vi "RMGetFrameCounters.vi"(0 "ResultManager":T1, 11 "error in (no error)":errorcluster) -> (3 "capturedFrames":i32, 4 "ResultManager (out)":T1, 6 "startFrame":i32, 8 "totalLocalizationsDone":i32, 10 "endFrame":i32, 13 "lostFrames":i32, 14 "lastSaveFrame":i32, 15 "error":errorcluster)   [LabVIEW 2011]
uses:
  ResultManagerInstance.ctl
  QTrkDLL.vi
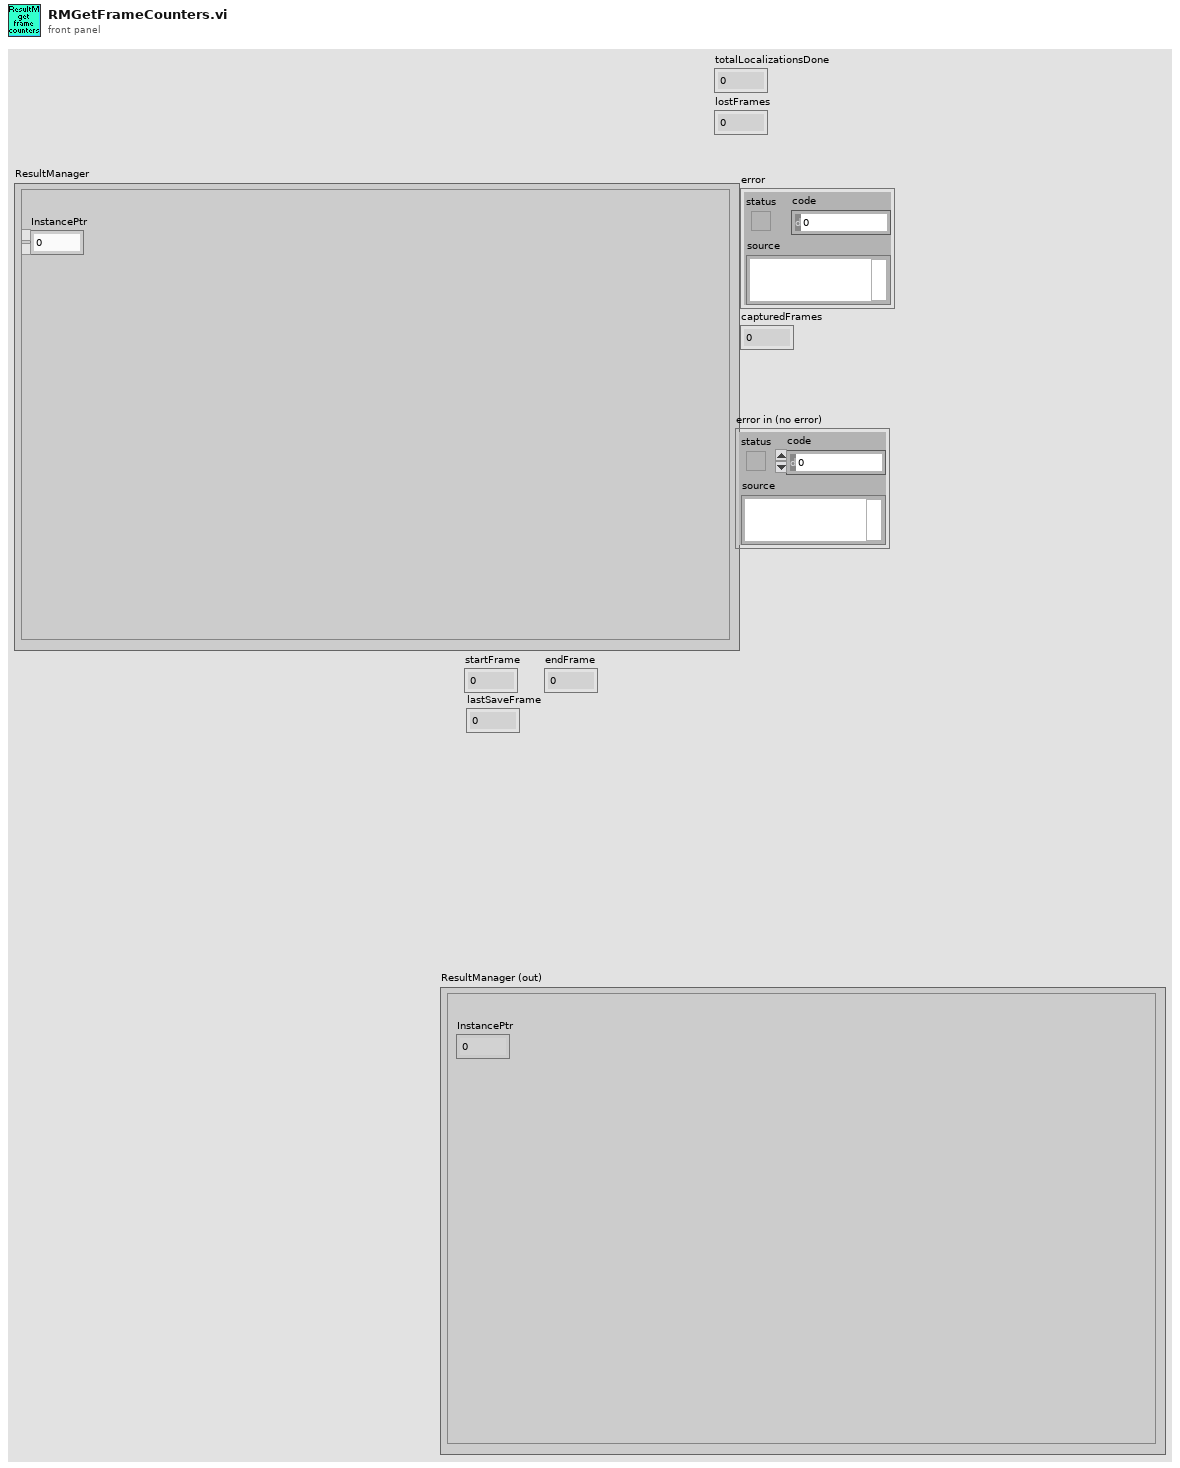
[diagram p1: front panel]
types:
  T1 = typedef "ResultManagerInstance.ctl" = cluster{"InstancePtr":u64}
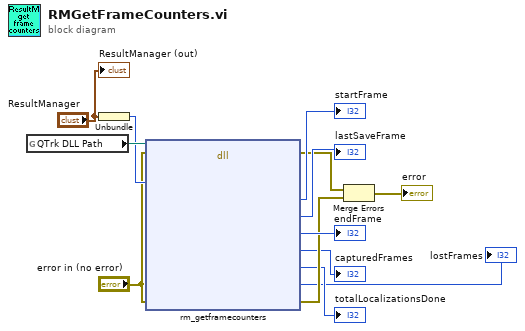
[diagram p0: block diagram]
diagram:
  n1 = global read "QTrkDLL.vi" "QTrk DLL Path"() -> (w13:path)
  n2 = Unbundle("ResultManager") -> ("InstancePtr"=w11:u64)
  n3 = dll-call lib="D:/jcnossen1/cudaqi-tracker/bin/jtrk-labview.dll" fn="rm_getframecounters"(path in=w13, error in="error in (no error)", "resultmanager"=w11, "err"="error in (no error)") -> (error out=w6:errorcluster, "startFrame"=→"startFrame":i32, "lastSaveFrame"=→"lastSaveFrame":i32, "endFrame"=→"endFrame":i32, "capturedFrames"=→"capturedFrames":i32, "totalLocalizationsDone"=→"totalLocalizationsDone":i32, "lostFrames"=→"lostFrames":i32, "err"=w5:errorcluster)  [unwired: 9 in, 1 out]
  n4 = Merge Errors(w6, w5) -> (→"error":errorcluster)
  "ResultManager (out)" <- "ResultManager"
